vi "pipequeue bench.vi"() -> ()   [LabVIEW 2013]
uses:
  protocol.ctl
  domain.ctl
  lvnano.lvlib
  <vilib>/addons/zeromq/zmq_context.lvclass
  <vilib>/addons/zeromq/socket_type.ctl
  <vilib>/addons/zeromq/zeromq.lvlib
  <vilib>/addons/zeromq/zmq_socket.lvclass
panel:
  out "LAST MSG":string
  out "exectime":dbl
  in  "messages":i32=1
  in  "size":i32=1024
  out "error out":errorcluster
  # "Z TCP:\n4.52/500k msg/1k size"
  # "nn tcp:\n7.87/5k msg/1M size"
  # "NN TCP:\n14.9288/500k msg/1k size"
  # "NN IPC:\n14.9288/500k msg/1k size"
  # "z tcp:\n9.2/5k msg/1M size"
  # "Nanomessage inproc:\n4.5/5k msg/1M size"
  # "Nanomessage inproc:\n7.93/500k msg/1k size"
  # "LVQ:\n0.396/5k msg/1M size"
  # "LVQ:\n0.521/500k msg/1k size"
  # "TCP:\n6.51435/5k msg/1M size"
  # "TCP:\n9.0131/500k msg/1k size"
  # "Z inproc:\n4.33/5k msg/1M size"
  # "Z inproc:\n4.69/500k msg/1k size"
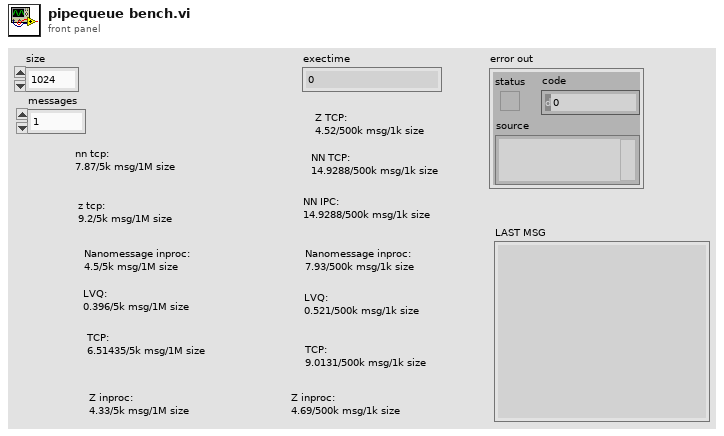
[diagram p1: front panel]
types:
  T1 = typedef "lvnano.lvlib/domain.ctl" = enum16{"Invalid", "AF_SP", "AF_SP_RAW"}
  T2 = typedef "zeromq.lvlib/socket_type.ctl" = enum8{"ZMQ_PAIR", "ZMQ_PUB", "ZMQ_SUB", "ZMQ_REQ", "ZMQ_REP", "ZMQ_DEALER", "ZMQ_ROUTER", "ZMQ_PULL", "ZMQ_PUSH", "ZMQ_XPUB", "ZMQ_XSUB"}
  T3 = typedef "lvnano.lvlib/protocol.ctl" = i32
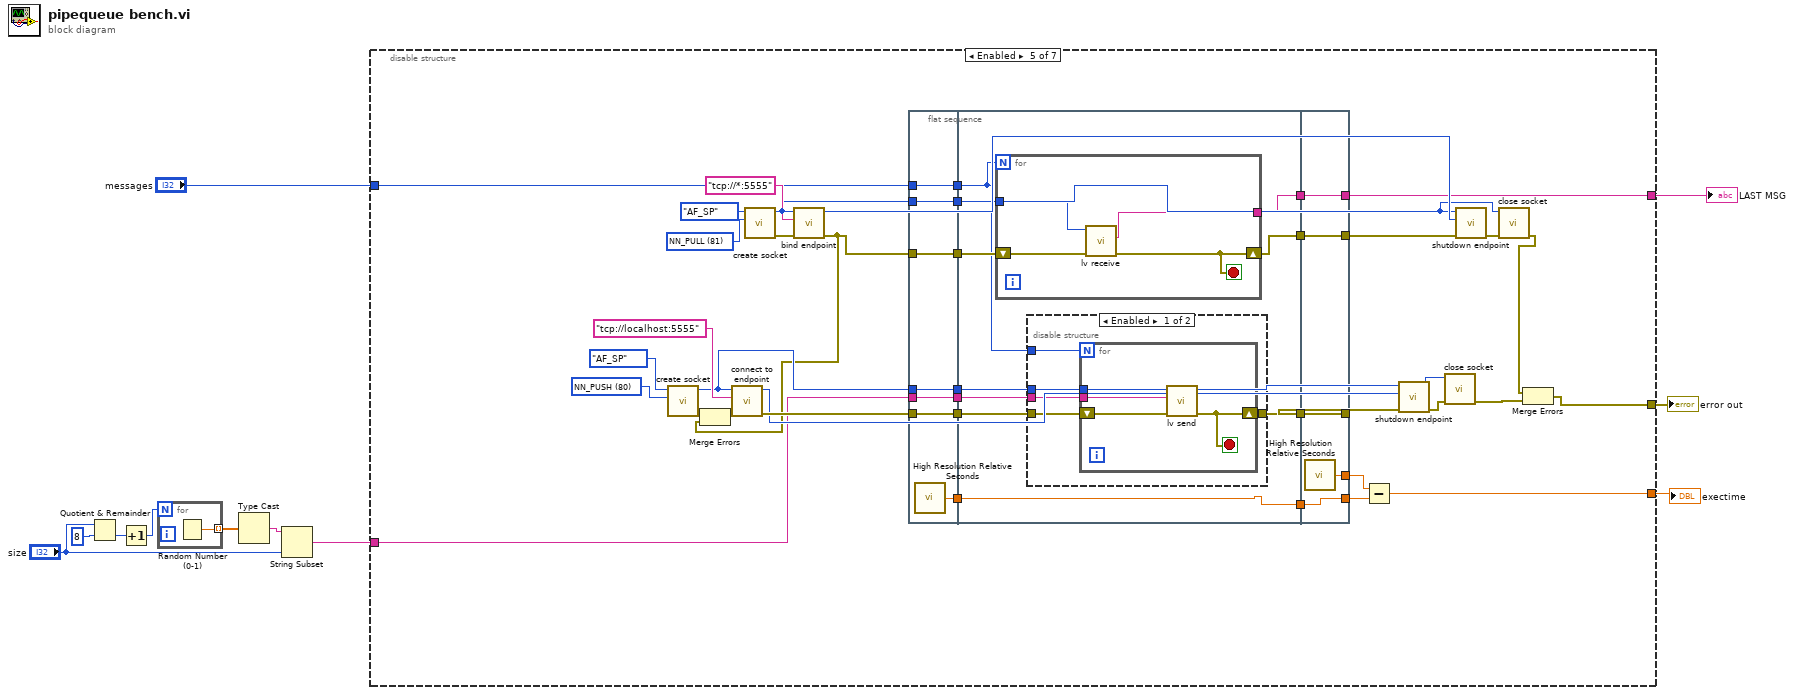
[diagram p0: block diagram]
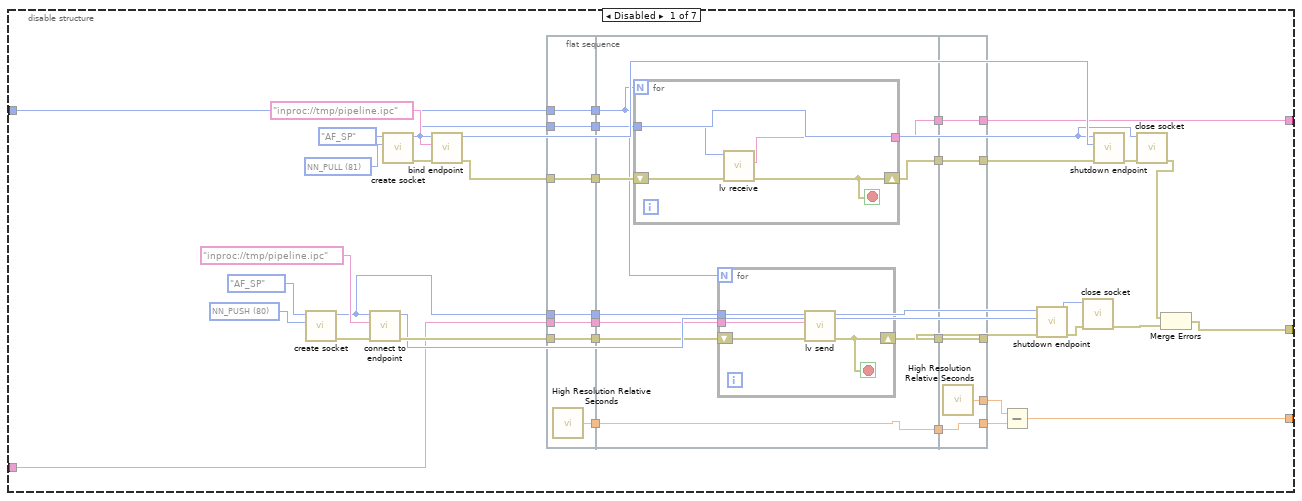
[diagram p2: hidden frame]
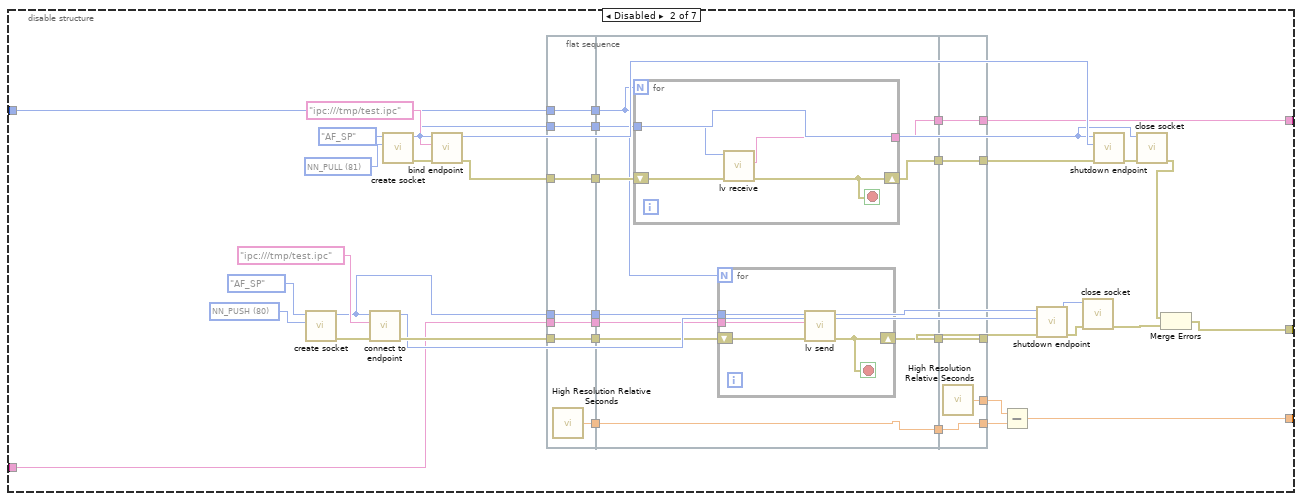
[diagram p3: hidden frame]
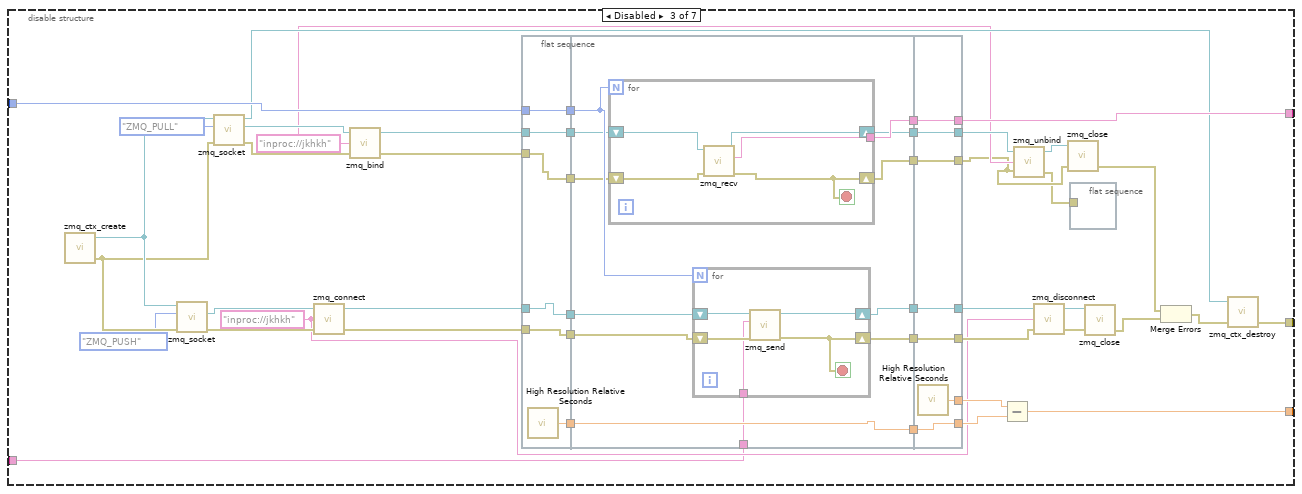
[diagram p4: hidden frame]
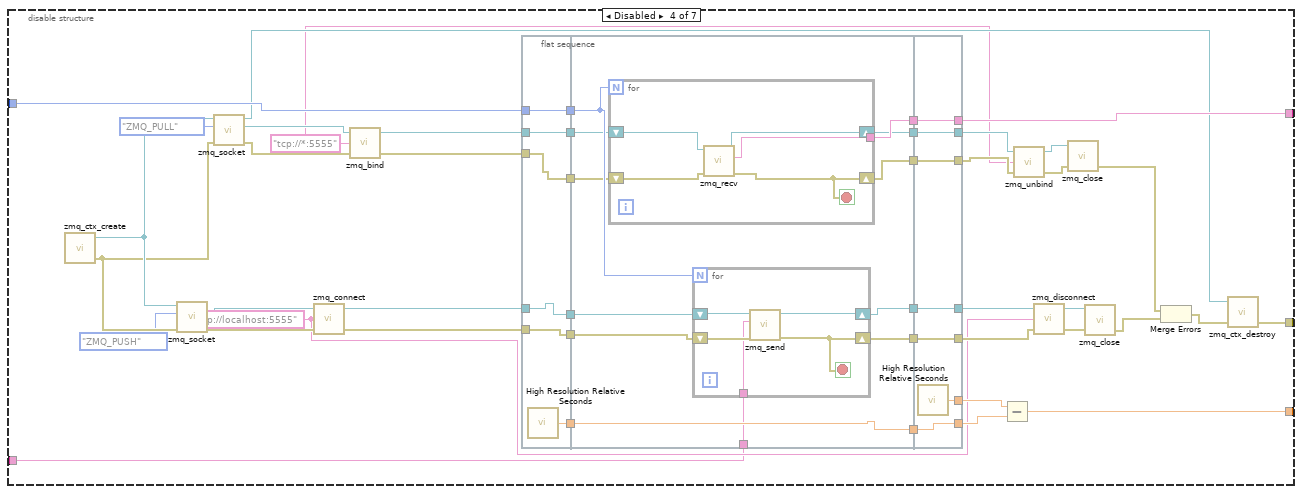
[diagram p5: hidden frame]
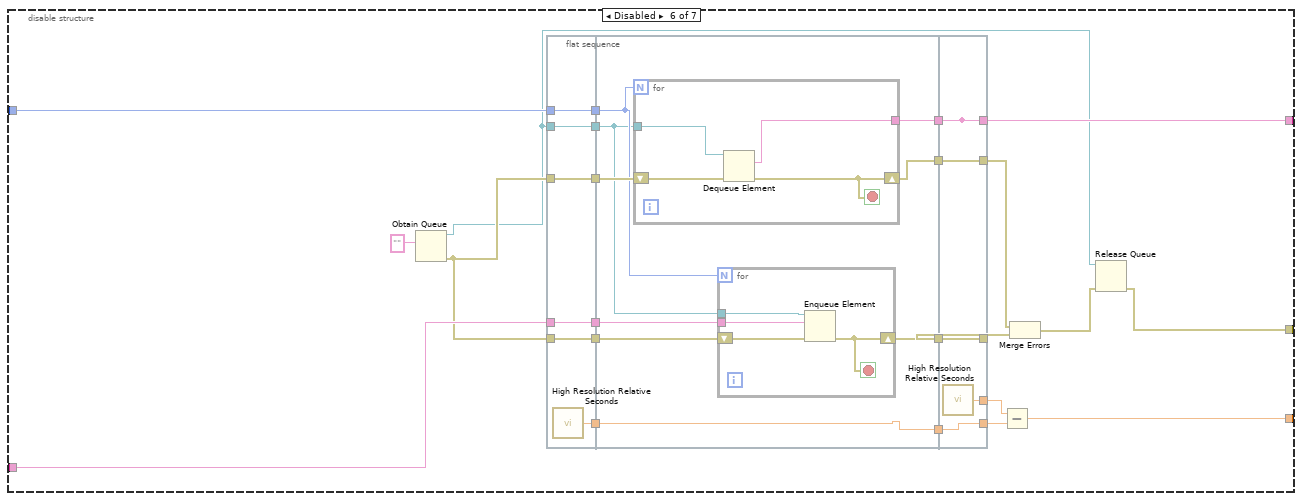
[diagram p7: hidden frame]
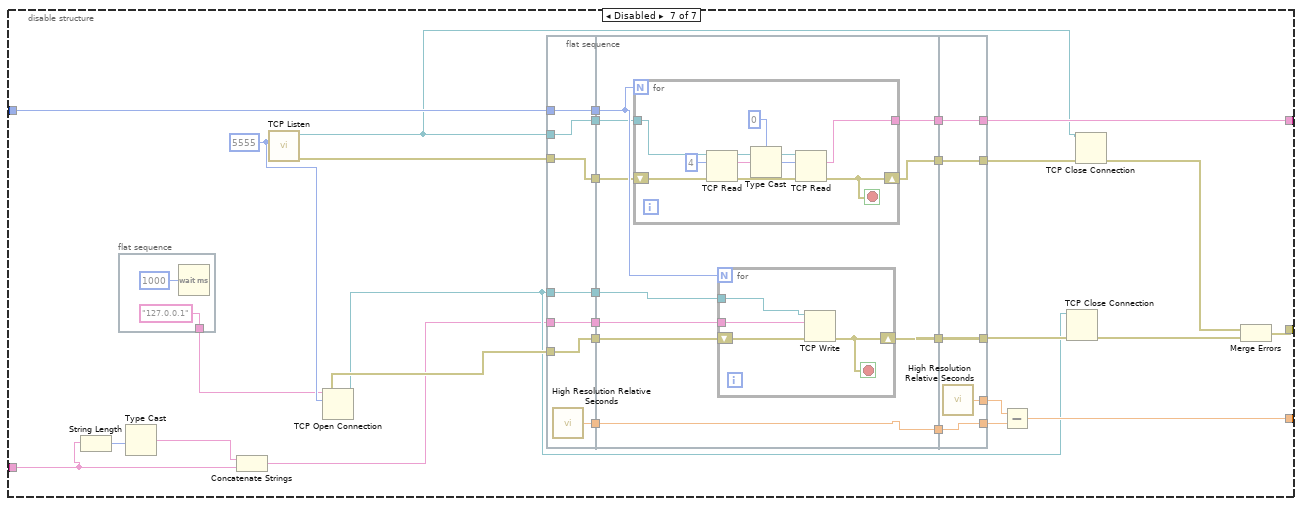
[diagram p8: hidden frame]
diagram:
  n1 = Quotient & Remainder(x="size", y=8) -> (floor(x/y)=w10:i32)  [unwired: 1 out]
  n2 = Increment(x=w10) -> (x+1=w8:i32)
  n3 = for {
    N: w8 -> [_]
    tunnel: [w12] -> w7 mode=indexing
    n4 = Random Number (0-1)() -> (number: 0 to 1=w12:dbl)
  }
  n5 = Type Cast(x=w7) -> (*(type *) &x=w6:string)  [unwired: 1 in]
  n6 = String Subset(string=w6, length (rest)="size") -> (substring=w3:string)  [unwired: 1 in]
  n7 = disable-structure shown="Enabled" {
    disable-tunnel: [w34 w102 w170 w248 w332 w384 w452] -> w11
    disable-tunnel: "messages" -> [w29 w97 w192 w272 w327 w406 w465]
    disable-tunnel: w3 -> [w28 w96 w151 w229 w326 w405 w438]
    disable-tunnel: [w15 w83 w184 w264 w313 w393 w456] -> w2
    disable-tunnel: [w13 w81 w182 w262 w311 w391 w454] -> w1
    frame Disabled {
      w45 = T3 80 items=["NN_PUSH"=80, "NN_PULL"=81] ("protocol")
      w48 = T3 81 items=["NN_PUSH"=80, "NN_PULL"=81] ("protocol")
      n8 = call "create socket.vi"("protocol"=w45, "domain"=domain."AF_SP") -> ("error out"=w43:errorcluster, "socket"=w38:i64)  [unwired: 8 in]
      n9 = call "connect to endpoint.vi"("error in"=w43, "address"="inproc://tmp/pipeline.ipc" ("addr"), "socket"=w38) -> ("error out"=w41:errorcluster, "endpoint"=w33:i32)  [unwired: 7 in]
      n10 = call "create socket.vi"("protocol"=w48, "domain"=domain."AF_SP") -> ("error out"=w50:errorcluster, "socket"=w31:i64)  [unwired: 8 in]
      n11 = call "bind endpoint.vi"("error in"=w50, "address"="inproc://tmp/pipeline.ipc" ("addr"), "socket"=w31) -> ("error out"=w46:errorcluster, "endpoint"=w32:i32)  [unwired: 7 in]
      n12 = flat-sequence {
        tunnel: w28 -> [w52]
        tunnel: w29 -> [w53]
        tunnel: w31 -> [w54]
        tunnel: w38 -> [w55]
        tunnel: w41 -> [w56]
        tunnel: w46 -> [w57]
        tunnel: [w57] -> w25
        tunnel: [w56] -> w24
        tunnel: [w55] -> w23
        tunnel: [w54] -> w22
        tunnel: [w53] -> w21
        tunnel: [w52] -> w20
        tunnel: [w51] -> w18
        tunnel: [w65] -> w27
        tunnel: [w62] -> w26
        tunnel: w25 -> [w67]
        tunnel: w24 -> [w66]
        tunnel: w23 -> [w64]
        tunnel: w22 -> [w63]
        tunnel: w21 -> [w59]
        tunnel: w20 -> [w61]
        tunnel: w18 -> [w60]
        tunnel: [w60] -> w17
        tunnel: [w58] -> w14
        tunnel: [w79] -> w30
        tunnel: [w80] -> w40
        tunnel: w27 -> [w80]
        tunnel: w26 -> [w79]
        tunnel: [w78] -> w19
        tunnel: w17 -> [w77]
        tunnel: [w77] -> w16
        tunnel: w14 -> [w76]
        tunnel: [w76] -> w13
        frame #0 {
          n13 = call <vilib>:"High Resolution Relative Seconds.vi"() -> ("relative seconds"=w51:dbl)
        }
        frame #1 {
          n14 = for {
            N: w59 -> [_]
            tunnel: w63 -> [w74]
            shift-right: [w73] -> w62
            shift-left: w67 -> [w75]
            tunnel: [w72] -> w58
            stop <- w73 stop-if-true
            n15 = call "lv receive.vi"("error in"=w75, "socket"=w74) -> ("error out"=w73:errorcluster, "data"=w72:string)  [unwired: 8 in]
          }
          n16 = for {
            N: w59 -> [_]
            tunnel: w61 -> [w70]
            tunnel: w64 -> [w69]
            shift-right: [w68] -> w65
            shift-left: w66 -> [w71]
            stop <- w68 stop-if-true
            n17 = call "lv send.vi"("error in"=w71, "data"=w70, "socket"=w69) -> ("error out"=w68:errorcluster)  [unwired: 8 in]
          }
        }
        frame #2 {
          n18 = call <vilib>:"High Resolution Relative Seconds.vi"() -> ("relative seconds"=w78:dbl)
        }
      }
      n19 = Subtract(x=w19, y=w16) -> (x-y=w15:dbl)
      n20 = call "shutdown endpoint.vi"("error in"=w40, "endpoint"=w33, "socket"=w38) -> ("error out"=w37:errorcluster)  [unwired: 8 in]
      n21 = call "close socket.vi"("error in"=w37, "socket"=w38) -> ("error out"=w35:errorcluster)  [unwired: 9 in]
      n22 = call "shutdown endpoint.vi"("error in"=w30, "endpoint"=w32, "socket"=w31) -> ("error out"=w39:errorcluster)  [unwired: 8 in]
      n23 = call "close socket.vi"("error in"=w39, "socket"=w31) -> ("error out"=w36:errorcluster)  [unwired: 9 in]
      n24 = Merge Errors(w36, w35) -> (w34:errorcluster)
    }
    frame Disabled {
      w113 = T3 80 items=["NN_PUSH"=80, "NN_PULL"=81] ("protocol")
      w116 = T3 81 items=["NN_PUSH"=80, "NN_PULL"=81] ("protocol")
      n25 = call "create socket.vi"("protocol"=w113, "domain"=domain."AF_SP") -> ("error out"=w111:errorcluster, "socket"=w106:i64)  [unwired: 8 in]
      n26 = call "connect to endpoint.vi"("error in"=w111, "address"="ipc:///tmp/test.ipc" ("addr"), "socket"=w106) -> ("error out"=w109:errorcluster, "endpoint"=w101:i32)  [unwired: 7 in]
      n27 = call "create socket.vi"("protocol"=w116, "domain"=domain."AF_SP") -> ("error out"=w118:errorcluster, "socket"=w99:i64)  [unwired: 8 in]
      n28 = call "bind endpoint.vi"("error in"=w118, "address"="ipc:///tmp/test.ipc" ("addr"), "socket"=w99) -> ("error out"=w114:errorcluster, "endpoint"=w100:i32)  [unwired: 7 in]
      n29 = flat-sequence {
        tunnel: w96 -> [w120]
        tunnel: w97 -> [w121]
        tunnel: w99 -> [w122]
        tunnel: w106 -> [w123]
        tunnel: w109 -> [w124]
        tunnel: w114 -> [w125]
        tunnel: [w125] -> w93
        tunnel: [w124] -> w92
        tunnel: [w123] -> w91
        tunnel: [w122] -> w90
        tunnel: [w121] -> w89
        tunnel: [w120] -> w88
        tunnel: [w119] -> w86
        tunnel: [w133] -> w95
        tunnel: [w130] -> w94
        tunnel: w93 -> [w135]
        tunnel: w92 -> [w134]
        tunnel: w91 -> [w132]
        tunnel: w90 -> [w131]
        tunnel: w89 -> [w127]
        tunnel: w88 -> [w129]
        tunnel: w86 -> [w128]
        tunnel: [w128] -> w85
        tunnel: [w126] -> w82
        tunnel: [w147] -> w98
        tunnel: [w148] -> w108
        tunnel: w95 -> [w148]
        tunnel: w94 -> [w147]
        tunnel: [w146] -> w87
        tunnel: w85 -> [w145]
        tunnel: [w145] -> w84
        tunnel: w82 -> [w144]
        tunnel: [w144] -> w81
        frame #0 {
          n30 = call <vilib>:"High Resolution Relative Seconds.vi"() -> ("relative seconds"=w119:dbl)
        }
        frame #1 {
          n31 = for {
            N: w127 -> [_]
            tunnel: w131 -> [w142]
            shift-right: [w141] -> w130
            shift-left: w135 -> [w143]
            tunnel: [w140] -> w126
            stop <- w141 stop-if-true
            n32 = call "lv receive.vi"("error in"=w143, "socket"=w142) -> ("error out"=w141:errorcluster, "data"=w140:string)  [unwired: 8 in]
          }
          n33 = for {
            N: w127 -> [_]
            tunnel: w129 -> [w138]
            tunnel: w132 -> [w137]
            shift-right: [w136] -> w133
            shift-left: w134 -> [w139]
            stop <- w136 stop-if-true
            n34 = call "lv send.vi"("error in"=w139, "data"=w138, "socket"=w137) -> ("error out"=w136:errorcluster)  [unwired: 8 in]
          }
        }
        frame #2 {
          n35 = call <vilib>:"High Resolution Relative Seconds.vi"() -> ("relative seconds"=w146:dbl)
        }
      }
      n36 = Subtract(x=w87, y=w84) -> (x-y=w83:dbl)
      n37 = call "shutdown endpoint.vi"("error in"=w108, "endpoint"=w101, "socket"=w106) -> ("error out"=w105:errorcluster)  [unwired: 8 in]
      n38 = call "close socket.vi"("error in"=w105, "socket"=w106) -> ("error out"=w103:errorcluster)  [unwired: 9 in]
      n39 = call "shutdown endpoint.vi"("error in"=w98, "endpoint"=w100, "socket"=w99) -> ("error out"=w107:errorcluster)  [unwired: 8 in]
      n40 = call "close socket.vi"("error in"=w107, "socket"=w99) -> ("error out"=w104:errorcluster)  [unwired: 9 in]
      n41 = Merge Errors(w104, w103) -> (w102:errorcluster)
    }
    frame Disabled {
      w152 = "inproc://jkhkh" ("endpoint")
      w153 = "inproc://jkhkh" ("endpoint")
      n42 = call <vilib>:"zmq_ctx_create.vi"() -> ("error out"=w180:errorcluster, "context out"=w181:refnum<class "zmq_context.lvclass">)  [unwired: 4 in]
      n43 = call <vilib>:"zmq_socket.vi"("error in"=w180, "socket type"=socket_type."ZMQ_PUSH", "context in"=w181) -> ("error out"=w166:errorcluster, "socket out"=w171:refnum<class "zmq_socket.lvclass">)  [unwired: 2 in, 1 out]
      n44 = call <vilib>:"zmq_socket.vi"("error in"=w180, "socket type"=socket_type."ZMQ_PULL", "context in"=w181) -> ("error out"=w161:errorcluster, "socket out"=w160:refnum<class "zmq_socket.lvclass">, "context out"=w169:refnum<class "zmq_context.lvclass">)  [unwired: 2 in]
      n45 = call <vilib>:"zmq_connect.vi"("error in"=w166, "endpoint"=w152, "socket in"=w171) -> ("error out"=w164:errorcluster, "socket out"=w162:refnum<class "zmq_socket.lvclass">)  [unwired: 1 in]
      n46 = call <vilib>:"zmq_bind.vi"("error in"=w161, "endpoint"=w153, "socket in"=w160) -> ("error out"=w154:errorcluster, "socket out"=w159:refnum<class "zmq_socket.lvclass">)  [unwired: 1 in]
      n47 = flat-sequence {
        tunnel: w192 -> [w199]
        tunnel: [w199] -> w189
        tunnel: [w198] -> w187
        tunnel: [w197] -> w165
        tunnel: w164 -> [w197]
        tunnel: [w196] -> w163
        tunnel: w162 -> [w196]
        tunnel: w159 -> [w195]
        tunnel: [w195] -> w158
        tunnel: [w194] -> w155
        tunnel: w154 -> [w194]
        tunnel: [w211] -> w191
        tunnel: [w210] -> w190
        tunnel: w189 -> [w208]
        tunnel: w187 -> [w209]
        tunnel: [w209] -> w186
        tunnel: [w207] -> w183
        tunnel: [w204] -> w168
        tunnel: w165 -> [w206]
        tunnel: w163 -> [w205]
        tunnel: w158 -> [w203]
        tunnel: [w202] -> w156
        tunnel: w155 -> [w201]
        tunnel: w151 -> [w200]
        tunnel: [w227] -> w150
        tunnel: [w228] -> w173
        tunnel: w191 -> [w228]
        tunnel: w190 -> [w227]
        tunnel: [w226] -> w188
        tunnel: w186 -> [w225]
        tunnel: [w225] -> w185
        tunnel: w183 -> [w224]
        tunnel: [w224] -> w182
        tunnel: w168 -> [w223]
        tunnel: [w223] -> w167
        tunnel: [w222] -> w157
        tunnel: w156 -> [w222]
        frame #0 {
          n48 = call <vilib>:"High Resolution Relative Seconds.vi"() -> ("relative seconds"=w198:dbl)
        }
        frame #1 {
          n49 = for {
            N: w208 -> [_]
            shift-right: [w218] -> w210
            shift-left: w201 -> [w221]
            tunnel: [w220] -> w207
            shift-right: [w219] -> w202
            shift-left: w203 -> [w217]
            stop <- w218 stop-if-true
            n50 = call <vilib>:"zmq_recv.vi"("error in"=w221, "socket in"=w217) -> ("error out"=w218:errorcluster, "data"=w220:string, "socket out"=w219:refnum<class "zmq_socket.lvclass">)  [unwired: 3 in, 2 out]
          }
          n51 = for {
            N: w208 -> [_]
            shift-right: [w214] -> w211
            shift-left: w206 -> [w213]
            shift-right: [w215] -> w204
            shift-left: w205 -> [w216]
            tunnel: w200 -> [w212]
            stop <- w214 stop-if-true
            n52 = call <vilib>:"zmq_send.vi"("error in"=w213, "data"=w212, "socket in"=w216) -> ("error out"=w214:errorcluster, "socket out"=w215:refnum<class "zmq_socket.lvclass">)  [unwired: 4 in]
          }
        }
        frame #2 {
          n53 = call <vilib>:"High Resolution Relative Seconds.vi"() -> ("relative seconds"=w226:dbl)
        }
      }
      n54 = Subtract(x=w188, y=w185) -> (x-y=w184:dbl)
      n55 = call <vilib>:"zmq_unbind.vi"("error in"=w150, "endpoint"=w153, "socket in"=w157) -> ("error out"=w149:errorcluster, "socket out"=w172:refnum<class "zmq_socket.lvclass">)  [unwired: 1 in]
      n56 = call <vilib>:"zmq_disconnect.vi"("error in"=w173, "endpoint"=w152, "socket in"=w167) -> ("error out"=w175:errorcluster, "socket out"=w174:refnum<class "zmq_socket.lvclass">)  [unwired: 1 in]
      n57 = call <vilib>:"zmq_close.vi"("error in"=w150, "socket"=w172) -> ("error out"=w176:errorcluster)  [unwired: 3 in]
      n58 = flat-sequence {
        tunnel: w149 -> [_]
        frame #0 {
        }
      }
      n59 = call <vilib>:"zmq_close.vi"("error in"=w175, "socket"=w174) -> ("error out"=w177:errorcluster)  [unwired: 3 in]
      n60 = Merge Errors(w176, w177) -> (w193:errorcluster)
      n61 = call <vilib>:"zmq_ctx_destroy.vi"("error in"=w193, "context in"=w169) -> ("error out"=w170:errorcluster)  [unwired: 3 in]
    }
    frame Disabled {
      w230 = "tcp://localhost:5555" ("endpoint")
      w231 = "tcp://*:5555" ("endpoint")
      n62 = call <vilib>:"zmq_ctx_create.vi"() -> ("error out"=w260:errorcluster, "context out"=w261:refnum<class "zmq_context.lvclass">)  [unwired: 4 in]
      n63 = call <vilib>:"zmq_socket.vi"("error in"=w260, "socket type"=socket_type."ZMQ_PUSH", "context in"=w261) -> ("error out"=w244:errorcluster, "socket out"=w249:refnum<class "zmq_socket.lvclass">)  [unwired: 2 in, 1 out]
      n64 = call <vilib>:"zmq_socket.vi"("error in"=w260, "socket type"=socket_type."ZMQ_PULL", "context in"=w261) -> ("error out"=w239:errorcluster, "socket out"=w238:refnum<class "zmq_socket.lvclass">, "context out"=w247:refnum<class "zmq_context.lvclass">)  [unwired: 2 in]
      n65 = call <vilib>:"zmq_connect.vi"("error in"=w244, "endpoint"=w230, "socket in"=w249) -> ("error out"=w242:errorcluster, "socket out"=w240:refnum<class "zmq_socket.lvclass">)  [unwired: 1 in]
      n66 = call <vilib>:"zmq_bind.vi"("error in"=w239, "endpoint"=w231, "socket in"=w238) -> ("error out"=w232:errorcluster, "socket out"=w237:refnum<class "zmq_socket.lvclass">)  [unwired: 1 in]
      n67 = flat-sequence {
        tunnel: w272 -> [w279]
        tunnel: [w279] -> w269
        tunnel: [w278] -> w267
        tunnel: [w277] -> w243
        tunnel: w242 -> [w277]
        tunnel: [w276] -> w241
        tunnel: w240 -> [w276]
        tunnel: w237 -> [w275]
        tunnel: [w275] -> w236
        tunnel: [w274] -> w233
        tunnel: w232 -> [w274]
        tunnel: [w291] -> w271
        tunnel: [w290] -> w270
        tunnel: w269 -> [w288]
        tunnel: w267 -> [w289]
        tunnel: [w289] -> w266
        tunnel: [w287] -> w263
        tunnel: [w284] -> w246
        tunnel: w243 -> [w286]
        tunnel: w241 -> [w285]
        tunnel: w236 -> [w283]
        tunnel: [w282] -> w234
        tunnel: w233 -> [w281]
        tunnel: w229 -> [w280]
        tunnel: [w307] -> w252
        tunnel: [w308] -> w253
        tunnel: w271 -> [w308]
        tunnel: w270 -> [w307]
        tunnel: [w306] -> w268
        tunnel: w266 -> [w305]
        tunnel: [w305] -> w265
        tunnel: w263 -> [w304]
        tunnel: [w304] -> w262
        tunnel: w246 -> [w303]
        tunnel: [w303] -> w245
        tunnel: [w302] -> w235
        tunnel: w234 -> [w302]
        frame #0 {
          n68 = call <vilib>:"High Resolution Relative Seconds.vi"() -> ("relative seconds"=w278:dbl)
        }
        frame #1 {
          n69 = for {
            N: w288 -> [_]
            shift-right: [w298] -> w290
            shift-left: w281 -> [w301]
            tunnel: [w300] -> w287
            shift-right: [w299] -> w282
            shift-left: w283 -> [w297]
            stop <- w298 stop-if-true
            n70 = call <vilib>:"zmq_recv.vi"("error in"=w301, "socket in"=w297) -> ("error out"=w298:errorcluster, "data"=w300:string, "socket out"=w299:refnum<class "zmq_socket.lvclass">)  [unwired: 3 in, 2 out]
          }
          n71 = for {
            N: w288 -> [_]
            shift-right: [w294] -> w291
            shift-left: w286 -> [w293]
            shift-right: [w295] -> w284
            shift-left: w285 -> [w296]
            tunnel: w280 -> [w292]
            stop <- w294 stop-if-true
            n72 = call <vilib>:"zmq_send.vi"("error in"=w293, "data"=w292, "socket in"=w296) -> ("error out"=w294:errorcluster, "socket out"=w295:refnum<class "zmq_socket.lvclass">)  [unwired: 4 in]
          }
        }
        frame #2 {
          n73 = call <vilib>:"High Resolution Relative Seconds.vi"() -> ("relative seconds"=w306:dbl)
        }
      }
      n74 = Subtract(x=w268, y=w265) -> (x-y=w264:dbl)
      n75 = call <vilib>:"zmq_unbind.vi"("error in"=w252, "endpoint"=w231, "socket in"=w235) -> ("error out"=w250:errorcluster, "socket out"=w251:refnum<class "zmq_socket.lvclass">)  [unwired: 1 in]
      n76 = call <vilib>:"zmq_disconnect.vi"("error in"=w253, "endpoint"=w230, "socket in"=w245) -> ("error out"=w255:errorcluster, "socket out"=w254:refnum<class "zmq_socket.lvclass">)  [unwired: 1 in]
      n77 = call <vilib>:"zmq_close.vi"("error in"=w250, "socket"=w251) -> ("error out"=w256:errorcluster)  [unwired: 3 in]
      n78 = call <vilib>:"zmq_close.vi"("error in"=w255, "socket"=w254) -> ("error out"=w257:errorcluster)  [unwired: 3 in]
      n79 = Merge Errors(w256, w257) -> (w273:errorcluster)
      n80 = call <vilib>:"zmq_ctx_destroy.vi"("error in"=w273, "context in"=w247) -> ("error out"=w248:errorcluster)  [unwired: 3 in]
    }
    frame Enabled {
      w343 = T3 80 items=["NN_PUSH"=80, "NN_PULL"=81] ("protocol")
      w345 = T3 81 items=["NN_PUSH"=80, "NN_PULL"=81] ("protocol")
      n81 = call "create socket.vi"("protocol"=w343, "domain"=domain."AF_SP") -> ("error out"=w341:errorcluster, "socket"=w336:i64)  [unwired: 8 in]
      n82 = call "create socket.vi"("protocol"=w345, "domain"=domain."AF_SP") -> ("error out"=w347:errorcluster, "socket"=w329:i64)  [unwired: 8 in]
      n83 = call "bind endpoint.vi"("error in"=w347, "address"="tcp://*:5555" ("addr"), "socket"=w329) -> ("error out"=w309:errorcluster, "endpoint"=w330:i32)  [unwired: 7 in]
      n84 = Merge Errors(w341, w309) -> (w310:errorcluster)
      n85 = call "connect to endpoint.vi"("error in"=w310, "address"="tcp://localhost:5555" ("addr"), "socket"=w336) -> ("error out"=w339:errorcluster, "endpoint"=w331:i32)  [unwired: 7 in]
      n86 = flat-sequence {
        tunnel: w326 -> [w349]
        tunnel: w327 -> [w350]
        tunnel: w329 -> [w351]
        tunnel: w336 -> [w352]
        tunnel: w339 -> [w353]
        tunnel: w309 -> [w354]
        tunnel: [w354] -> w323
        tunnel: [w353] -> w322
        tunnel: [w352] -> w321
        tunnel: [w351] -> w320
        tunnel: [w350] -> w319
        tunnel: [w349] -> w318
        tunnel: [w348] -> w316
        tunnel: [w362] -> w325
        tunnel: [w359] -> w324
        tunnel: w323 -> [w364]
        tunnel: w322 -> [w363]
        tunnel: w321 -> [w361]
        tunnel: w320 -> [w360]
        tunnel: w319 -> [w356]
        tunnel: w318 -> [w358]
        tunnel: w316 -> [w357]
        tunnel: [w357] -> w315
        tunnel: [w355] -> w312
        tunnel: [w382] -> w328
        tunnel: [w383] -> w338
        tunnel: w325 -> [w383]
        tunnel: w324 -> [w382]
        tunnel: [w381] -> w317
        tunnel: w315 -> [w380]
        tunnel: [w380] -> w314
        tunnel: w312 -> [w379]
        tunnel: [w379] -> w311
        frame #0 {
          n87 = call <vilib>:"High Resolution Relative Seconds.vi"() -> ("relative seconds"=w348:dbl)
        }
        frame #1 {
          n88 = for {
            N: w356 -> [_]
            tunnel: w360 -> [w377]
            shift-right: [w376] -> w359
            shift-left: w364 -> [w378]
            tunnel: [w375] -> w355
            stop <- w376 stop-if-true
            n89 = call "lv receive.vi"("error in"=w378, "socket"=w377) -> ("error out"=w376:errorcluster, "data"=w375:string)  [unwired: 8 in]
          }
          n90 = disable-structure shown="Enabled" {
            disable-tunnel: w363 -> [w369 w374]
            disable-tunnel: [w368 w374] -> w362
            disable-tunnel: w361 -> [w367 _]
            disable-tunnel: w358 -> [w366 _]
            disable-tunnel: w356 -> [w365 _]
            frame Enabled {
              n91 = for {
                N: w365 -> [_]
                tunnel: w366 -> [w372]
                tunnel: w367 -> [w371]
                shift-right: [w370] -> w368
                shift-left: w369 -> [w373]
                stop <- w370 stop-if-true
                n92 = call "lv send.vi"("error in"=w373, "data"=w372, "socket"=w371) -> ("error out"=w370:errorcluster)  [unwired: 8 in]
              }
            }
            frame Disabled {
            }
          }
        }
        frame #2 {
          n93 = call <vilib>:"High Resolution Relative Seconds.vi"() -> ("relative seconds"=w381:dbl)
        }
      }
      n94 = Subtract(x=w317, y=w314) -> (x-y=w313:dbl)
      n95 = call "shutdown endpoint.vi"("error in"=w338, "endpoint"=w331, "socket"=w336) -> ("error out"=w335:errorcluster)  [unwired: 8 in]
      n96 = call "close socket.vi"("error in"=w335, "socket"=w336) -> ("error out"=w333:errorcluster)  [unwired: 9 in]
      n97 = call "shutdown endpoint.vi"("error in"=w328, "endpoint"=w330, "socket"=w329) -> ("error out"=w337:errorcluster)  [unwired: 8 in]
      n98 = call "close socket.vi"("error in"=w337, "socket"=w329) -> ("error out"=w334:errorcluster)  [unwired: 9 in]
      n99 = Merge Errors(w334, w333) -> (w332:errorcluster)
    }
    frame Disabled {
      n100 = Obtain Queue(element data type="") -> (queue out=w387:refnum<queue>, error out=w389:errorcluster)  [unwired: 4 in, 1 out]
      n101 = flat-sequence {
        tunnel: w405 -> [w408]
        tunnel: w406 -> [w409]
        tunnel: w387 -> [w410]
        tunnel: w389 -> [w411]
        tunnel: w389 -> [w412]
        tunnel: [w412] -> w402
        tunnel: [w411] -> w401
        tunnel: [w410] -> w400
        tunnel: [w409] -> w399
        tunnel: [w408] -> w398
        tunnel: [w407] -> w396
        tunnel: [w419] -> w404
        tunnel: [w418] -> w403
        tunnel: w402 -> [w421]
        tunnel: w401 -> [w420]
        tunnel: w400 -> [w413]
        tunnel: w399 -> [w415]
        tunnel: w398 -> [w417]
        tunnel: w396 -> [w416]
        tunnel: [w416] -> w395
        tunnel: [w414] -> w392
        tunnel: [w433] -> w385
        tunnel: [w434] -> w388
        tunnel: w404 -> [w434]
        tunnel: w403 -> [w433]
        tunnel: [w432] -> w397
        tunnel: w395 -> [w431]
        tunnel: [w431] -> w394
        tunnel: [w430] -> _
        tunnel: w392 -> [w430]
        tunnel: [w430] -> w391
        frame #0 {
          n102 = call <vilib>:"High Resolution Relative Seconds.vi"() -> ("relative seconds"=w407:dbl)
        }
        frame #1 {
          n103 = for {
            N: w415 -> [_]
            tunnel: w413 -> [w428]
            shift-right: [w427] -> w418
            shift-left: w421 -> [w429]
            tunnel: [w426] -> w414
            stop <- w427 stop-if-true
            n104 = Dequeue Element(queue=w428, error in (no error)=w429) -> (element=w426:string, error out=w427:errorcluster)  [unwired: 1 in, 2 out]
          }
          n105 = for {
            N: w415 -> [_]
            tunnel: w417 -> [w424]
            shift-right: [w423] -> w419
            shift-left: w420 -> [w425]
            tunnel: w413 -> [w422]
            stop <- w423 stop-if-true
            n106 = Enqueue Element(queue=w422, element=w424, error in (no error)=w425) -> (error out=w423:errorcluster)  [unwired: 1 in, 2 out]
          }
        }
        frame #2 {
          n107 = call <vilib>:"High Resolution Relative Seconds.vi"() -> ("relative seconds"=w432:dbl)
        }
      }
      n108 = Subtract(x=w397, y=w394) -> (x-y=w393:dbl)
      n109 = Merge Errors(w385, w388) -> (w386:errorcluster)
      n110 = Release Queue(queue=w387, error in (no error)=w386) -> (error out=w384:errorcluster)  [unwired: 1 in, 2 out]
    }
    frame Disabled {
      w451 = u16 5555 ("port")
      n111 = String Length(string=w438) -> (length=w437:i32)
      n112 = flat-sequence {
        tunnel: ["127.0.0.1" ("address")] -> w439
        frame #0 {
          n113 = Wait (ms)(milliseconds to wait=u32 1000) -> ()  [unwired: 1 out]
        }
      }
      n114 = Type Cast(x=w437) -> (*(type *) &x=w435:string)  [unwired: 1 in]
      n115 = Concatenate Strings(w435, w438) -> (w436:string)
      n116 = call <vilib>:"TCP Listen.vi"("port"=w451) -> ("error out"=w445:errorcluster, "connection ID"=w441:refnum<k5>)  [unwired: 6 in, 3 out]
      n117 = TCP Open Connection(address=w439, remote port or service name=w451) -> (connection ID=w440:refnum<k5>, error out=w444:errorcluster)  [unwired: 3 in]
      n118 = flat-sequence {
        tunnel: w436 -> [w473]
        tunnel: w465 -> [w474]
        tunnel: [w474] -> w462
        tunnel: [w473] -> w461
        tunnel: [w472] -> w459
        tunnel: [w471] -> w447
        tunnel: w441 -> [w471]
        tunnel: [w470] -> w446
        tunnel: w445 -> [w470]
        tunnel: w444 -> [w469]
        tunnel: [w469] -> w443
        tunnel: [w468] -> w442
        tunnel: w440 -> [w468]
        tunnel: [w484] -> w464
        tunnel: [w483] -> w463
        tunnel: w462 -> [w480]
        tunnel: w461 -> [w482]
        tunnel: w459 -> [w481]
        tunnel: [w481] -> w458
        tunnel: [w479] -> w455
        tunnel: w447 -> [w478]
        tunnel: w446 -> [w477]
        tunnel: w443 -> [w476]
        tunnel: w442 -> [w475]
        tunnel: [w502] -> w450
        tunnel: [w503] -> w453
        tunnel: w464 -> [w503]
        tunnel: w463 -> [w502]
        tunnel: [w501] -> w460
        tunnel: w458 -> [w500]
        tunnel: [w500] -> w457
        tunnel: w455 -> [w499]
        tunnel: [w499] -> w454
        frame #0 {
          n119 = call <vilib>:"High Resolution Relative Seconds.vi"() -> ("relative seconds"=w472:dbl)
        }
        frame #1 {
          n120 = for {
            N: w480 -> [_]
            shift-right: [w497] -> w483
            shift-left: w477 -> [w498]
            tunnel: [w496] -> w479
            tunnel: w478 -> [w494]
            stop <- w497 stop-if-true
            n121 = TCP Read(connection ID=w494, bytes to read=4, error in (no error)=w498) -> (connection ID out=w493:refnum<k5>, data out=w491:string, error out=w495:errorcluster)  [unwired: 2 in]
            n122 = Type Cast(type=0, x=w491) -> (*(type *) &x=w490:i32)
            n123 = TCP Read(connection ID=w493, bytes to read=w490, error in (no error)=w495) -> (data out=w496:string, error out=w497:errorcluster)  [unwired: 2 in, 1 out]
          }
          n124 = for {
            N: w480 -> [_]
            tunnel: w482 -> [w487]
            shift-right: [w486] -> w484
            shift-left: w476 -> [w488]
            tunnel: w475 -> [w485]
            stop <- w486 stop-if-true
            n125 = TCP Write(connection ID=w485, data in=w487, error in (no error)=w488) -> (error out=w486:errorcluster)  [unwired: 1 in, 2 out]
          }
        }
        frame #2 {
          n126 = call <vilib>:"High Resolution Relative Seconds.vi"() -> ("relative seconds"=w501:dbl)
        }
      }
      n127 = Subtract(x=w460, y=w457) -> (x-y=w456:dbl)
      n128 = TCP Close Connection(connection ID=w440, error in (no error)=w453) -> (error out=w448:errorcluster)  [unwired: 1 in, 1 out]
      n129 = TCP Close Connection(connection ID=w441, error in (no error)=w450) -> (error out=w449:errorcluster)  [unwired: 1 in, 1 out]
      n130 = Merge Errors(w449, w448) -> (w452:errorcluster)
    }
  }
  "error out" <- w11
  "exectime" <- w2
  "LAST MSG" <- w1
